vi "SDSU_InitGeometry.vi"(0 "refnum":i32=2048, 1 "override format":string, 11 "error in (no error)":errorcluster, 12 "Database RefNum out":T1) -> (4 "fd out":i32, 6 "return value":i32, 8 "X total size":u16, 10 "Y total size":u16, 14 "DET_READ_TIME":sgl=3.5 format="%.6f", 15 "error out":errorcluster)   [LabVIEW 2016]
uses:
  DBSHAND/private/vis/DatabaseHand_RefNum.ctl
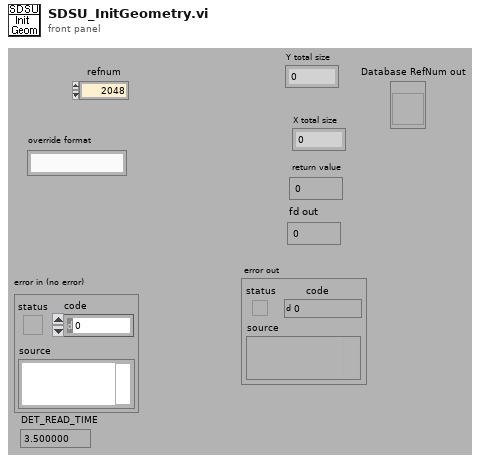
[diagram p1: front panel]
types:
  T1 = typedef "DatabaseHand_RefNum.ctl" = refnum<vi>
  T2 = cluster{"Video Processor Type":string, "support gain":bool, "Timing Board":string, "support reset":bool, "Utility Board":string, "Shutter":string, "Temperature":string, "support temp control":bool, "Detector Type":string, "Support MPP":string, "Support Binning":string, "Readout Mode":string, "support shutter control":bool}
  T3 = typedef "GEOM_CorrectedFPA.ctl" = cluster{"readmode":string, "amplifiers":cluster{"number":i32, "xstart":i32, "ystart":i32}[], "totxsize":i32, "totysize":i32, "maxxdim":i32, "maxydim":i32, "numxamps":i32, "numyamps":i32, "totxdata":i32, "totydata":i32, "xdataamp":i32, "ydataamp":i32, "totpixels":i32}
  T4 = typedef "GEOM_Amplifier.ctl" = cluster{"number":i32, "type":T5, "rotated":i16, "fliped":u16, "FPAcoord":cluster{"xstart":i32, "ystart":i32}, "Physical_size":cluster{"columns":i32, "rows":i32}, "predata":cluster{"columns":i32, "rows":i32}, "postdata":cluster{"columns":i32, "rows":i32}, "Req ROIs":T6, "Corr ROI":T6, "Detnumber":i32, "ampID":string, "discard":i32}
  T5 = typedef "GEOM_AmpType.ctl" = u16
  T6 = typedef "GEOM_ROI.ctl" = T7[]
  T7 = typedef "GEOM_Coords.ctl" = cluster{"xstart":u32, "ystart":u32, "xsize":u32, "ysize":u32}
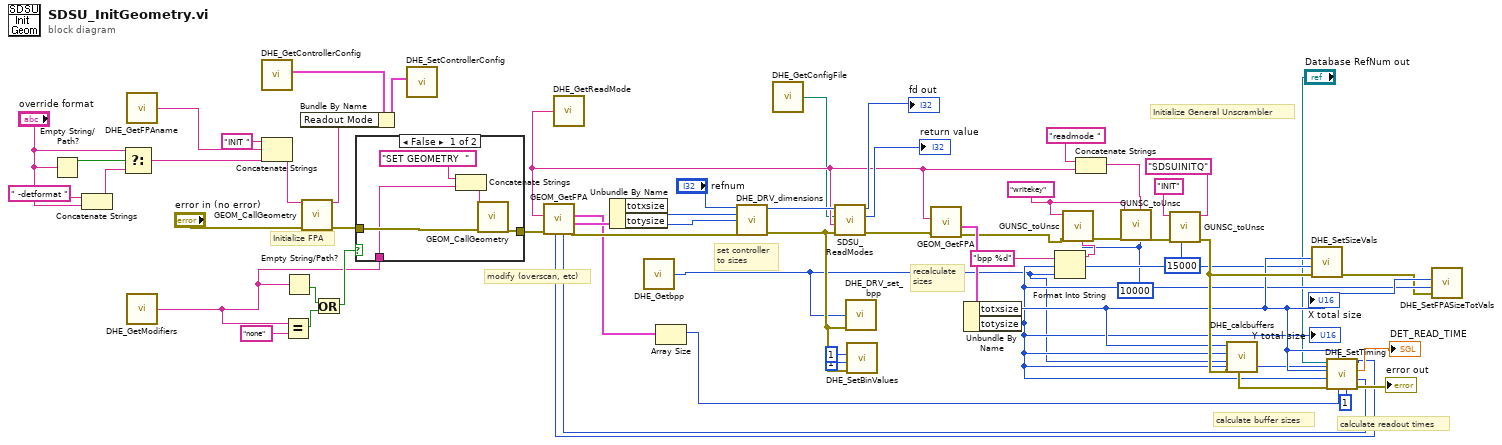
[diagram p0: block diagram]
diagram:
  w2 = 10000 ("ms timeout (-1)")
  w30 = "writekey" ("command")
  # "calculate readout times"
  # "calculate buffer sizes"
  # "Initialize General Unscrambler"
  # "recalculate\nsizes"
  # "set controller\nto sizes"
  # "modify (overscan, etc)"
  # "Initialize FPA"
  n1 = Empty String/Path?(string/path="override format") -> (empty?=w12:bool)
  n2 = Concatenate Strings(" -detformat " ("string"), "override format") -> (w8:string)
  n3 = Select(t="override format", s=w12, f=w8) -> (s? t:f=w11:string)
  n4 = call "DHE_GetFPAname.vi"() -> ("DHE_FPAname"=w7:string)  [unwired: 9 out]
  n5 = call "DHE_GetModifiers.vi"() -> ("DHE_Modifiers"=w6:string)  [unwired: 9 out]
  n6 = call "DHE_GetControllerConfig.vi"() -> ("ControllerConfigCluster"=w58:T2)  [unwired: 11 out]
  n7 = Concatenate Strings("INIT " ("string"), w7, w11) -> (w59:string)
  n8 = Equal?(x=w6, y="none") -> (x = y?=w34:bool)
  n9 = Empty String/Path?(string/path=w6) -> (empty?=w35:bool)
  n10 = call "GEOM_CallGeometry.vi"("Command"=w59, "error in (no error)"="error in (no error)") -> ("ImmedReplyString"=w57:string, "error out"=w55:errorcluster)  [unwired: 12 out]
  n11 = Bundle By Name(cluster=w58, "Readout Mode"=w57) -> (w56:T2)
  n12 = Or(x=w35, y=w34) -> (x .or. y?=w33:bool)
  n13 = case shown="False" w33 {
    tunnel: w55 -> [w65 w66]
    tunnel: [w62 w66] -> w54
    tunnel: w6 -> [w61 _]
    frame False {
      n14 = Concatenate Strings("SET GEOMETRY  " ("Command"), w61) -> (w63:string)
      n15 = call "GEOM_CallGeometry.vi"("Command"=w63, "error in (no error)"=w65) -> ("error out"=w62:errorcluster)  [unwired: 13 out]
    }
    frame True {
    }
  }
  n16 = call "DHE_SetControllerConfig.vi"("ControllerConfigCluster"=w56) -> ()  [unwired: 11 out]
  n17 = call "DHE_GetReadMode.vi"() -> ("DHE_ReadMode"=w5:string)  [unwired: 9 out]
  n18 = call "GEOM_GetFPA.vi"("error in (no error)"=w54, "readmode"=w5) -> ("error out"=w52:errorcluster, "CorrectedFPACoord"=w51:T3, "amplifiers"=w20:T4[], "numyamps"=w17:i32, "numxamps"=w18:i32)  [unwired: 1 in, 4 out]
  n19 = Unbundle By Name(w51) -> ("totxsize"=w38:i32, "totysize"=w39:i32)
  n20 = call "DHE_Getbpp.vi"() -> ("DHE_bpp"=w4:i32)  [unwired: 9 out]
  n21 = Array Size(array=w20) -> (size(s)=w28:i32)
  n22 = call "DHE_DRV_dimensions.vi"("fd"="refnum", "Columns"=w38, "Rows"=w39, "error in (no error)"=w52) -> ("fd out"=w21:i32, "error out"=w25:errorcluster)  [unwired: 10 out]
  n23 = call "DHE_GetConfigFile.vi"() -> ("DHE_ConfigFile"=w3:path)  [unwired: 9 out]
  n24 = call "SDSU_ReadModes.vi"("error in (no error)"=w25, "read mode"=w5, "configuration file path"=w3, "fd"=w21) -> ("error out"=w24:errorcluster, "error_code"=→"return value":i32, "fd out"=→"fd out":i32)  [unwired: 5 out]
  n25 = call "DHE_DRV_set_bpp.vi"("bpp"=w4, "error in (no error)"=w25) -> ()  [unwired: 1 in, 13 out]
  n26 = call "DHE_SetBinValues.vi"("error in"=w25, "ybin"=1, "xbin"=1) -> ()  [unwired: 9 out]
  n27 = call "GEOM_GetFPA.vi"("error in (no error)"=w24, "readmode"=w5) -> ("error out"=w32:errorcluster, "CorrectedFPACoord"=w40:T3)  [unwired: 1 in, 7 out]
  n28 = Unbundle By Name(w40) -> ("totxsize"=w16:i32, "totysize"=w15:i32)
  "Y total size" <- w15
  "X total size" <- w16
  n29 = Format Into String(format string="bpp %d", w4) -> (resulting string=w29:string)  [unwired: 2 in, 1 out]
  n30 = call "GUNSC_toUnsc.vi"("ms timeout (-1)"=w2, "key"=w29, "error in (no error)"=w32, "command"=w30) -> ("error out"=w31:errorcluster)  [unwired: 5 in, 2 out]
  n31 = Concatenate Strings("readmode " ("string"), w5) -> (w46:string)
  n32 = call "GUNSC_toUnsc.vi"("ms timeout (-1)"=w2, "key"=w46, "error in (no error)"=w31, "command"=w30) -> ("error out"=w49:errorcluster)  [unwired: 5 in, 2 out]
  n33 = call "GUNSC_toUnsc.vi"("responseQ"="SDSUINITQ", "bpp"=u32 15000, "error in (no error)"=w49, "command"="INIT") -> ("error out"=w37:errorcluster)  [unwired: 5 in, 2 out]
  n34 = call "DHE_calcbuffers.vi"("error in (no error)"=w37, "bpp"=w4, "nrows"=w15, "ncols"=w16) -> ("error out"=w43:errorcluster)  [unwired: 2 in, 5 out]
  n35 = call "DHE_SetSizeVals.vi"("error in"=w37, "ytotsize"=w15, "xtotsize"=w16) -> ("errorout"=w14:errorcluster)  [unwired: 8 out]
  n36 = call "DHE_SetTiming.vi"("num of Y amps"=w17, "num of X amps"=w18, "yroi start"=1, "roi rows"=w15, "Num of amps"=w28, "roi cols"=w16, "error in"=w43, "totysize"=w15, "totxsize"=w16, "Database RefNum out"="Database RefNum out") -> ("errorout"=→"error out":errorcluster, "DET_READ_TIME"=→"DET_READ_TIME":sgl)
  n37 = call "DHE_SetFPASizeTotVals.vi"("error in"=w14, "ytotsize"=w15, "xtotsize"=w16) -> ()  [unwired: 9 out]
